vi "Set Ctrl Colour.vi"(8 "error in (no error)":errorcluster, 9 "Inner Color":u32(colorbox), 10 "Outer Color":u32(colorbox), 11 "Ctrl Reference's in":refnum<class "Ctrl Reference's.lvclass">) -> (0 "error out":errorcluster, 3 "Ctrl Reference's out":refnum<class "Ctrl Reference's.lvclass">)   [LabVIEW 2020, in "Ctrl Reference's.lvclass"]
uses:
  Ctrl Reference's.lvclass
  Ctrl Reference's.lvclass/Ctrl Reference's.ctl
panel:
  in  "appended array":cluster{"Outer Color":u32, "Inner Color":u32}[](array[cluster])
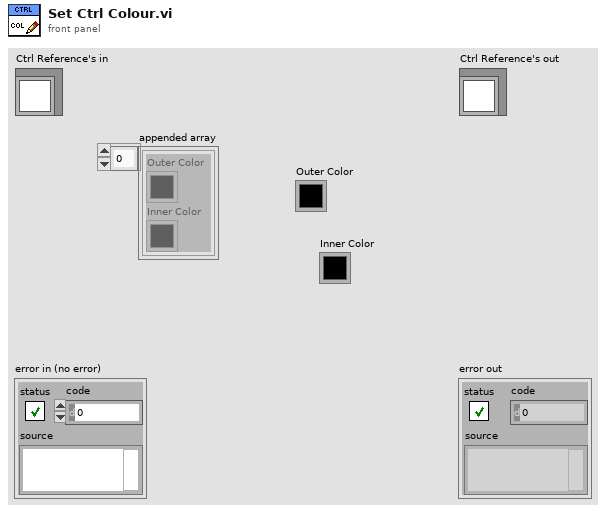
[diagram p1: front panel]
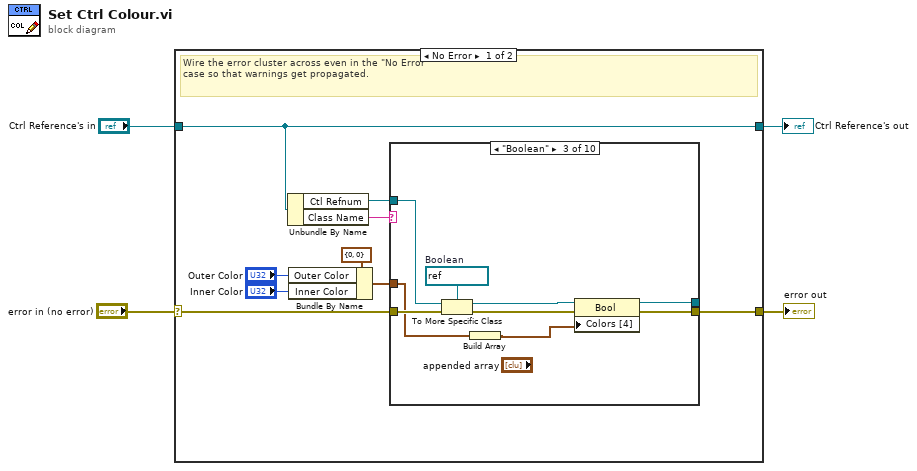
[diagram p0: block diagram]
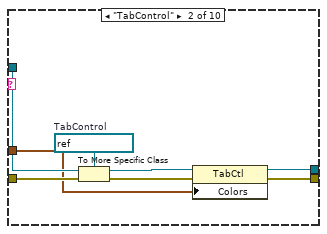
[diagram p3: hidden frame]
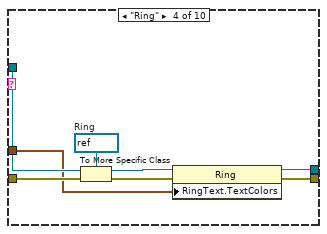
[diagram p4: hidden frame]
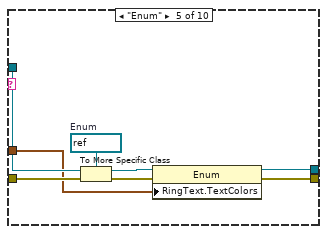
[diagram p5: hidden frame]
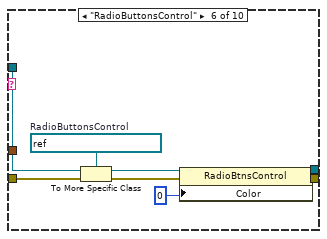
[diagram p6: hidden frame]
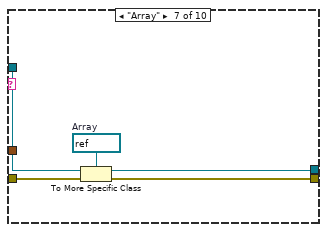
[diagram p7: hidden frame]
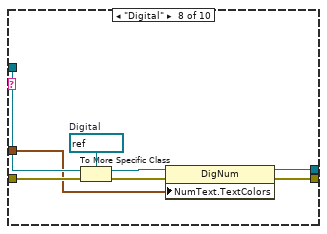
[diagram p8: hidden frame]
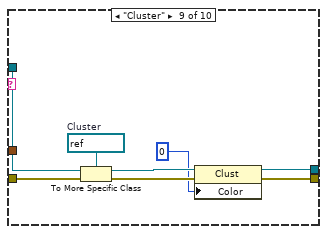
[diagram p9: hidden frame]
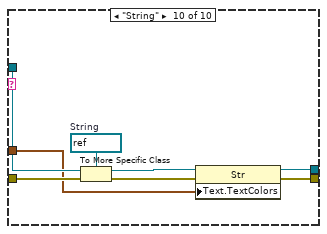
[diagram p10: hidden frame]
diagram:
  n1 = case shown="No Error" "error in (no error)" {
    selector: "error in (no error)" -> [w8 w84]
    tunnel: [w5 w84] -> w3
    tunnel: [w11 w83] -> w1
    tunnel: "Ctrl Reference's in" -> [w11 w83]
    frame No Error {
      # "Wire the error cluster across even in the \"No Error\"\ncase so that warnings get propagated."
      n2 = Unbundle By Name(w11) -> ("Ctl Refnum"=w10:refnum<vi>, "Class Name"=w9:string)
      n3 = Bundle By Name(cluster=cluster{"Outer Color":u32, "Inner Color":u32} {"Outer Color"=0, "Inner Color"=0} ("Color"), "Outer Color"="Outer Color", "Inner Color"="Inner Color") -> (w12:cluster{"Outer Color":u32, "Inner Color":u32})
      n4 = case shown="\"Boolean\"" w9 {
        tunnel: w8 -> [w14 w22 w31 w39 w47 w53 w58 w66 w74 w82]
        tunnel: w10 -> [_ w21 w30 w38 w46 w52 w57 w65 w73 w81]
        tunnel: [_ w16 w25 w32 w40 w49 w54 w59 w67 w76] -> _
        tunnel: [w14 w15 w26 w33 w41 w50 w55 w60 w68 w77] -> w5
        tunnel: w12 -> [_ w18 w24 w34 w42 _ _ w61 _ w75]
        frame Default {
        }
        frame "TabControl" {
          w20 = refnum<vi> refnum  # TabControl
          n5 = To More Specific Class(target class=w20, reference=w21, error in=w22) -> (specific class reference=w19:refnum<vi>, error out=w17:errorcluster)
          n6 = property class="TabCtl"(reference=w19, error in=w17, "Colors"=w18) -> (reference out=w16:refnum<vi>, error out=w15:errorcluster)
        }
        frame "Boolean" {
          w29 = refnum<vi> refnum  # Boolean
          n7 = To More Specific Class(target class=w29, reference=w30, error in=w31) -> (specific class reference=w28:refnum<vi>, error out=w27:errorcluster)
          n8 = Build Array(w24) -> (w23:cluster{"Outer Color":u32, "Inner Color":u32}[])
          n9 = property class="Bool"(reference=w28, error in=w27, "Colors [4]"=w23) -> (reference out=w25:refnum<vi>, error out=w26:errorcluster)
        }
        frame "Ring" {
          w37 = refnum<vi> refnum  # Ring
          n10 = To More Specific Class(target class=w37, reference=w38, error in=w39) -> (specific class reference=w35:refnum<vi>, error out=w36:errorcluster)
          n11 = property class="Ring"(reference=w35, error in=w36, "RingText.TextColors"=w34) -> (reference out=w32:refnum<vi>, error out=w33:errorcluster)
        }
        frame "Enum" {
          w45 = refnum<vi> refnum  # Enum
          n12 = To More Specific Class(target class=w45, reference=w46, error in=w47) -> (specific class reference=w43:refnum<vi>, error out=w44:errorcluster)
          n13 = property class="Enum"(reference=w43, error in=w44, "RingText.TextColors"=w42) -> (reference out=w40:refnum<vi>, error out=w41:errorcluster)
        }
        frame "RadioButtonsControl" {
          w51 = refnum<vi> refnum  # RadioButtonsControl
          n14 = To More Specific Class(target class=w51, reference=w52, error in=w53) -> (specific class reference=w49:refnum<vi>, error out=w50:errorcluster)
          n15 = property class="RadioBtnsControl"(reference=w49, error in=w50, "Color"=u32 0) -> ()  [unwired: 2 out]
        }
        frame "Array" {
          w56 = refnum<vi> refnum  # Array
          n16 = To More Specific Class(target class=w56, reference=w57, error in=w58) -> (specific class reference=w54:refnum<vi>, error out=w55:errorcluster)
        }
        frame "Digital" {
          w64 = refnum<vi> refnum  # Digital
          n17 = To More Specific Class(target class=w64, reference=w65, error in=w66) -> (specific class reference=w62:refnum<vi>, error out=w63:errorcluster)
          n18 = property class="DigNum"(reference=w62, error in=w63, "NumText.TextColors"=w61) -> (reference out=w59:refnum<vi>, error out=w60:errorcluster)
        }
        frame "Cluster" {
          w72 = refnum<vi> refnum  # Cluster
          n19 = To More Specific Class(target class=w72, reference=w73, error in=w74) -> (specific class reference=w71:refnum<vi>, error out=w70:errorcluster)
          n20 = property class="Clust"(reference=w71, error in=w70, "Color"=u32 0) -> (reference out=w67:refnum<vi>, error out=w68:errorcluster)
        }
        frame "String" {
          w80 = refnum<vi> refnum  # String
          n21 = To More Specific Class(target class=w80, reference=w81, error in=w82) -> (specific class reference=w78:refnum<vi>, error out=w79:errorcluster)
          n22 = property class="Str"(reference=w78, error in=w79, "Text.TextColors"=w75) -> (reference out=w76:refnum<vi>, error out=w77:errorcluster)
        }
      }
    }
    frame Error {
    }
  }
  "error out" <- w3
  "Ctrl Reference's out" <- w1
